vi "Create Event References.vi"(8 "error in":errorcluster) -> (0 "error out":errorcluster, 3 "ase":T1)   [LabVIEW 2024, in "serenial.io-ase.lvlib" / "ase.lvclass"]
doc: "<B>Create the Standard Output, Standard Error and Did Exit event references.</B>"
uses:
  ase.lvclass
  Event References.ctl
  Standard Output.ctl
  Standard Error.ctl
  Did Exit.ctl
  ase.lvclass/ase.ctl
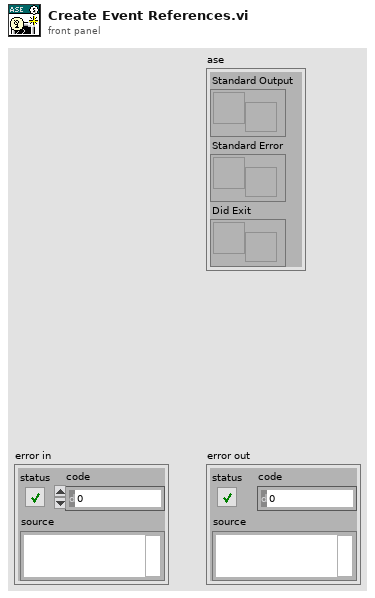
[diagram p1: front panel]
types:
  T1 = typedef "serenial.io-ase.lvlib/ase.lvclass/Event References.ctl" = cluster{"Standard Output":refnum<user-event>, "Standard Error":refnum<user-event>, "Did Exit":refnum<user-event>}
  T2 = typedef "serenial.io-ase.lvlib/ase.lvclass/Did Exit.ctl" = cluster{"Exit Code":i32, "ID":string}
  T3 = typedef "serenial.io-ase.lvlib/ase.lvclass/Standard Error.ctl" = cluster{"Data":string, "ID":string}
  T4 = typedef "serenial.io-ase.lvlib/ase.lvclass/Standard Output.ctl" = cluster{"Data":string, "ID":string}
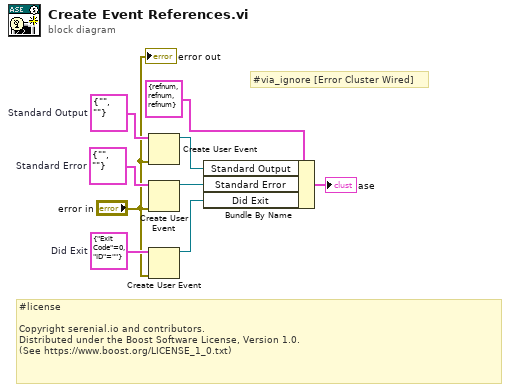
[diagram p0: block diagram]
diagram:
  w7 = T2 {"Exit Code"=0, "ID"=""}  # Did Exit
  w5 = T3 {"Data"="", "ID"=""}  # Standard Error
  w3 = T4 {"Data"="", "ID"=""}  # Standard Output
  # "#license\n\nCopyright serenial.io and contributors.\nDistributed under the Boost Software License, Version 1.0.\n(See https://www.boost.org/LICENSE_1_0.txt)"
  # "#via_ignore [Error Cluster Wired]"
  n1 = Create User Event(user event datatype=w3, error in="error in") -> (user event=w2:refnum<user-event>)  [unwired: 1 out]
  n2 = Create User Event(user event datatype=w5, error in="error in") -> (user event=w4:refnum<user-event>)  [unwired: 1 out]
  n3 = Create User Event(user event datatype=w7, error in="error in") -> (user event=w6:refnum<user-event>)  [unwired: 1 out]
  n4 = Bundle By Name(cluster=T1 {"Standard Output"=refnum, "Standard Error"=refnum, "Did Exit"=refnum} ("Event References"), "Standard Output"=w2, "Standard Error"=w4, "Did Exit"=w6) -> (→"ase":T1)
  "error out" <- "error in"
